vi "Add Device.vi"(8 "error in (no error)":errorcluster, 11 "Configuration Editor in":refnum<class "Configuration Editor.lvclass">) -> (0 "error out":errorcluster, 3 "Configuration Editor out":refnum<class "Configuration Editor.lvclass">)   [LabVIEW 2023, in "Configuration Editor.lvlib" / "Configuration Editor.lvclass"]
uses:
  Library/Configuration Editor.lvclass
  Library/Configuration Editor.lvclass/Configuration Editor.ctl
  builds/Framework/Configuration.lvlibp/Library/Configuration.lvclass
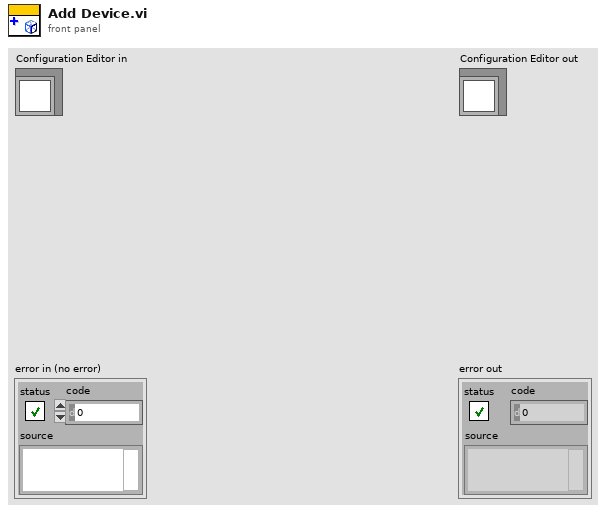
[diagram p1: front panel]
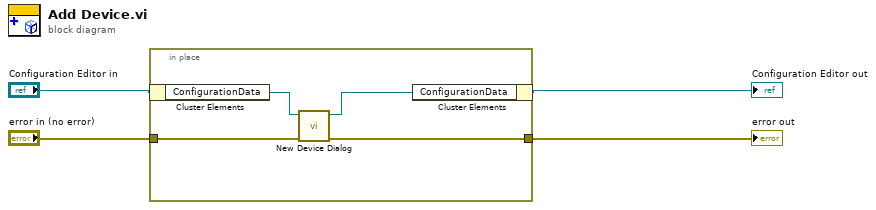
[diagram p0: block diagram]
diagram:
  n1 = in-place {
    in-place-border: "error in (no error)" -> [w6]
    in-place-border: [w5] -> w1
    n2 = in-place-cluster #1("Configuration Editor in") -> ("ConfigurationData"=w8:refnum<class "Configuration.lvclass">)
    n3 = call "New Device Dialog.vi"("error in (no error)"=w6, "Configuration in"=w8) -> ("error out"=w5:errorcluster, "Configuration out"=w7:refnum<class "Configuration.lvclass">)  [unwired: 6 in, 2 out]
    n4 = in-place-cluster #1("ConfigurationData"=w7) -> (→"Configuration Editor out":refnum<class "Configuration Editor.lvclass">)
  }
  "error out" <- w1
